vi "(TestVI)Waveform Editor Tree UI.vi"() -> ()   [LabVIEW 2020]
panel:
  in  "트리 2":string[](tree)
  in  "WF Seq":i32[](listbox)
  in  "WF List":i32[](listbox)
  in  "트리":string(tree)
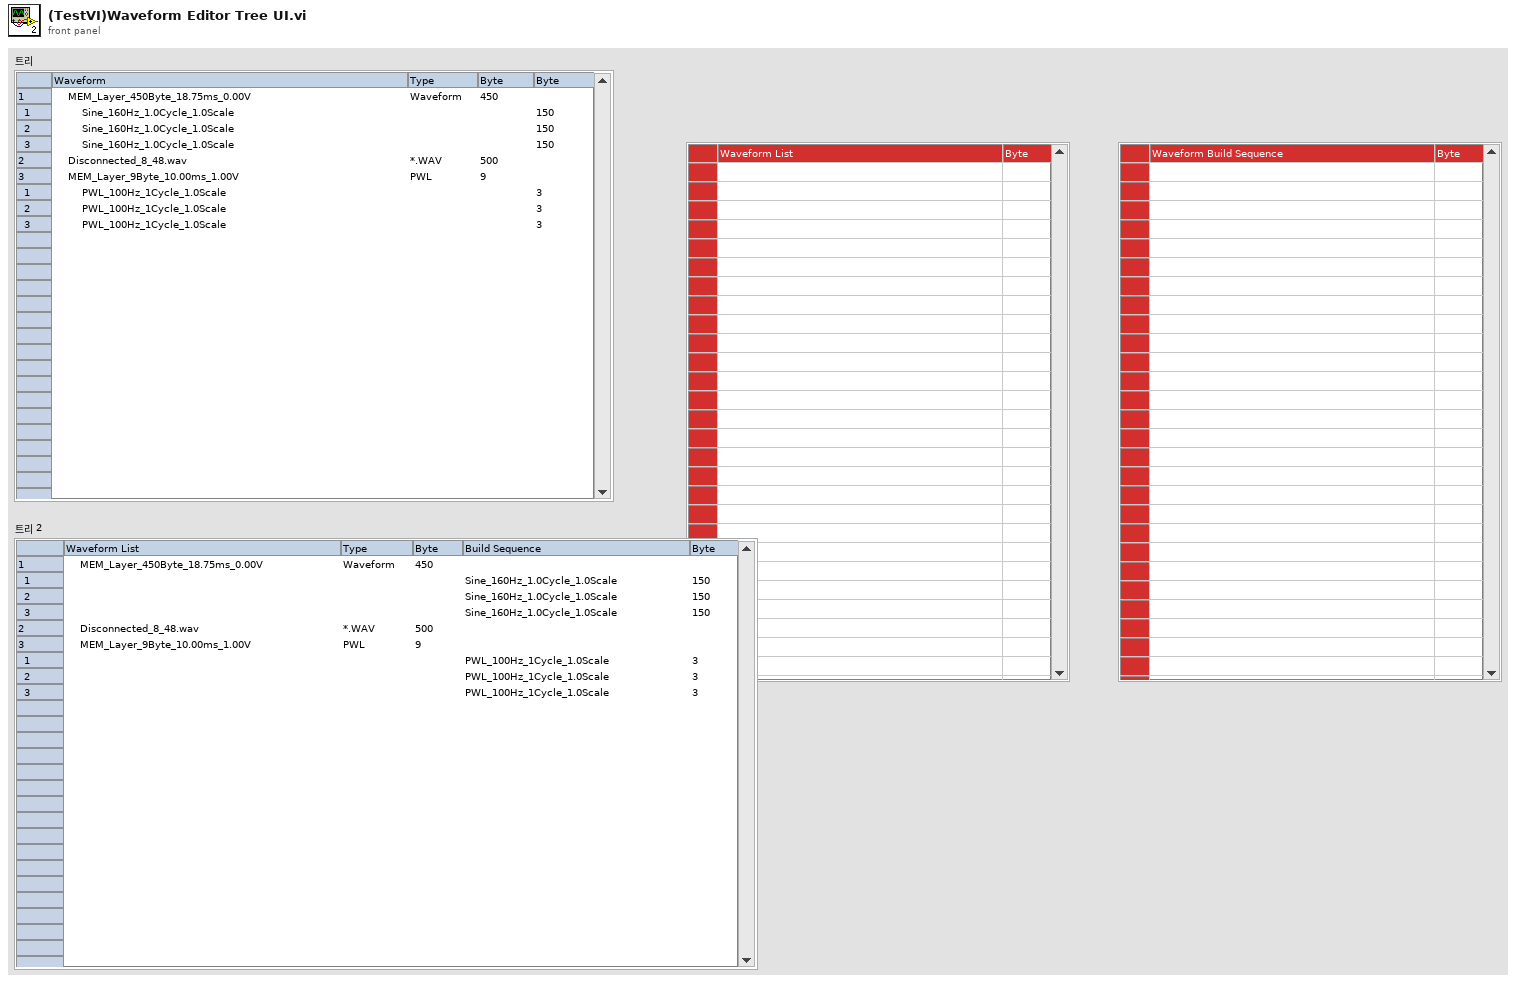
[diagram p1: front panel]
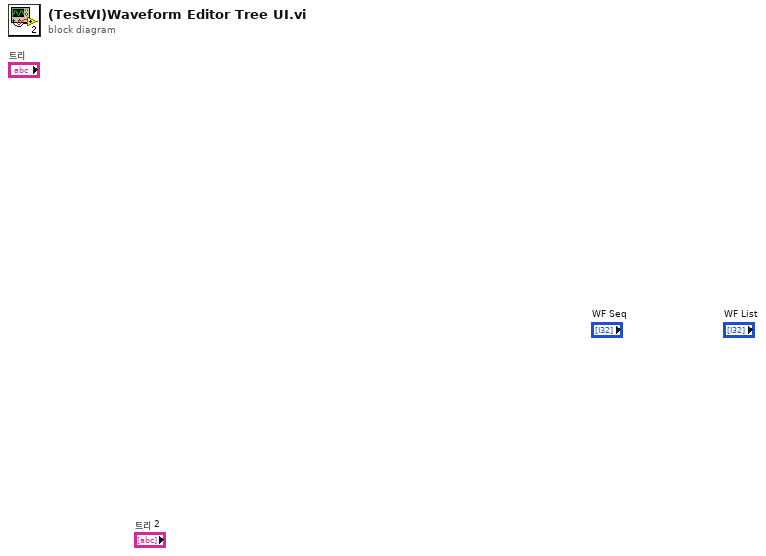
[diagram p0: block diagram]
diagram:
